vi "stft_demodulate_low.vi"(6 "Reset":bool, 9 "Config":T3={"IO params"={"Conversion"={"Rate"=4.0, "Num cards"=2, "Out channels"=4}, "Carriers"={"Phase shift"=180.0, "Levels"=[[0.8, 0.8, 0.8], [0.03, 0.03, 0.03]], "Delay samples"=73.15}, "TCP"={"Host"="192.168.1.15", "Port"=6666, "Buffering"=6, "Timeout"=6}, "Input channel sign"=[1, 1, 1]}, "High rate STFT"={"Win param"=101.5, "Window type"=61, "Win order"=2, "DFT size"=64, "Channels"=[7], "Oversample"=64}, "Low rate STFT"={"Win param"=120.0, "Window type"=61, "Win order"=8, "DFT size"=64, "Channels"=[7], "Oversample"=64}, "Filtering "=[]} {"Filtering"."Distortion"."Limit" format="%#_3p"; "Filtering"."Distortion"."LF cut" format="%#_3p"; "Filtering"."Kalman"."Measure noise" format="%#_3p"; "Filtering"."Kalman"."Process noise" format="%#_3p"; "Filtering"."Hum"."Limit" format="%#_3p"; "Filtering"."Hum"."Frequency" format="%#_4p"; "Low rate STFT"."Oversample" min=1 step=1; "Low rate STFT"."Channels" min=0 step=1; "Low rate STFT"."DFT size" min=1 step=1; "Low rate STFT"."Window type" items=["Rectangle"=0, "Hanning"=1, "Hamming"=2, "Blackman-Harris"=3, "Exact Blackman"=4, "Blackman"=5, "Flat Top"=6, "4 Term B-Harris "=7, "7 Term B-Harris"=8, "Low Sidelobe"=9, "Blackman Nuttall"=11, "Triangle"=30, "Bartlett-Hanning"=31, "Bohman"=32, "Parzen"=33, "Welch"=34, "Kaiser"=60, "Dolph-Chebyshev"=61, "Gaussian"=62]; "High rate STFT"."Oversample" min=1 step=1; "High rate STFT"."Channels" min=0 step=1; "High rate STFT"."DFT size" min=1 step=1; "High rate STFT"."Window type" items=["Rectangle"=0, "Hanning"=1, "Hamming"=2, "Blackman-Harris"=3, "Exact Blackman"=4, "Blackman"=5, "Flat Top"=6, "4 Term B-Harris "=7, "7 Term B-Harris"=8, "Low Sidelobe"=9, "Blackman Nuttall"=11, "Triangle"=30, "Bartlett-Hanning"=31, "Bohman"=32, "Parzen"=33, "Welch"=34, "Kaiser"=60, "Dolph-Chebyshev"=61, "Gaussian"=62]; "IO params"."Input channel sign" min=-1 max=1 step=1; "IO params"."Carriers"."Levels" min=0.0 step=0.1; "IO params"."Conversion"."Rate" format="%#_8g"}, 10 "Modulation info":T2={"Fs full"=0.0, "Fs high"=0.0, "Fs low"=0.0, "Read size"=0, "FFT size low"=5000, "df low"=5000.0, "High carriers"=[], "Low carriers"=[], "Hi channels at low"=[7]} {"Hi channels at low" min=0 step=1; "Low carriers" format="%#_6p"; "High carriers" format="%#_6p"}, 11 "Raw data":dbl[][](array[numeric])) -> (2 "STFT":cdb[][](array[numeric]) format="%#_4p", 3 "Card carrier amplitudes":T1 format="%#_3p")   [LabVIEW 2026]
uses:
  ilemt_config.ctl
  system/IO_params.ctl
  stft_params.ctl
  <vilib>/Analysis/4window.llb/windowTd.ctl
  filter_params.ctl
  detrend_mode.ctl
  modulation_info.ctl
  card_carrier_amplitudes.ctl
  <vilib>/Analysis/NI_AALPro.lvlib
panel:
  # "The demodulated carrier amplitudes (a coupling matrix) . The page index is high/low."
  # "Each row is the complex spectrum for the XYZ input channels.  This gets stored in the trace info."
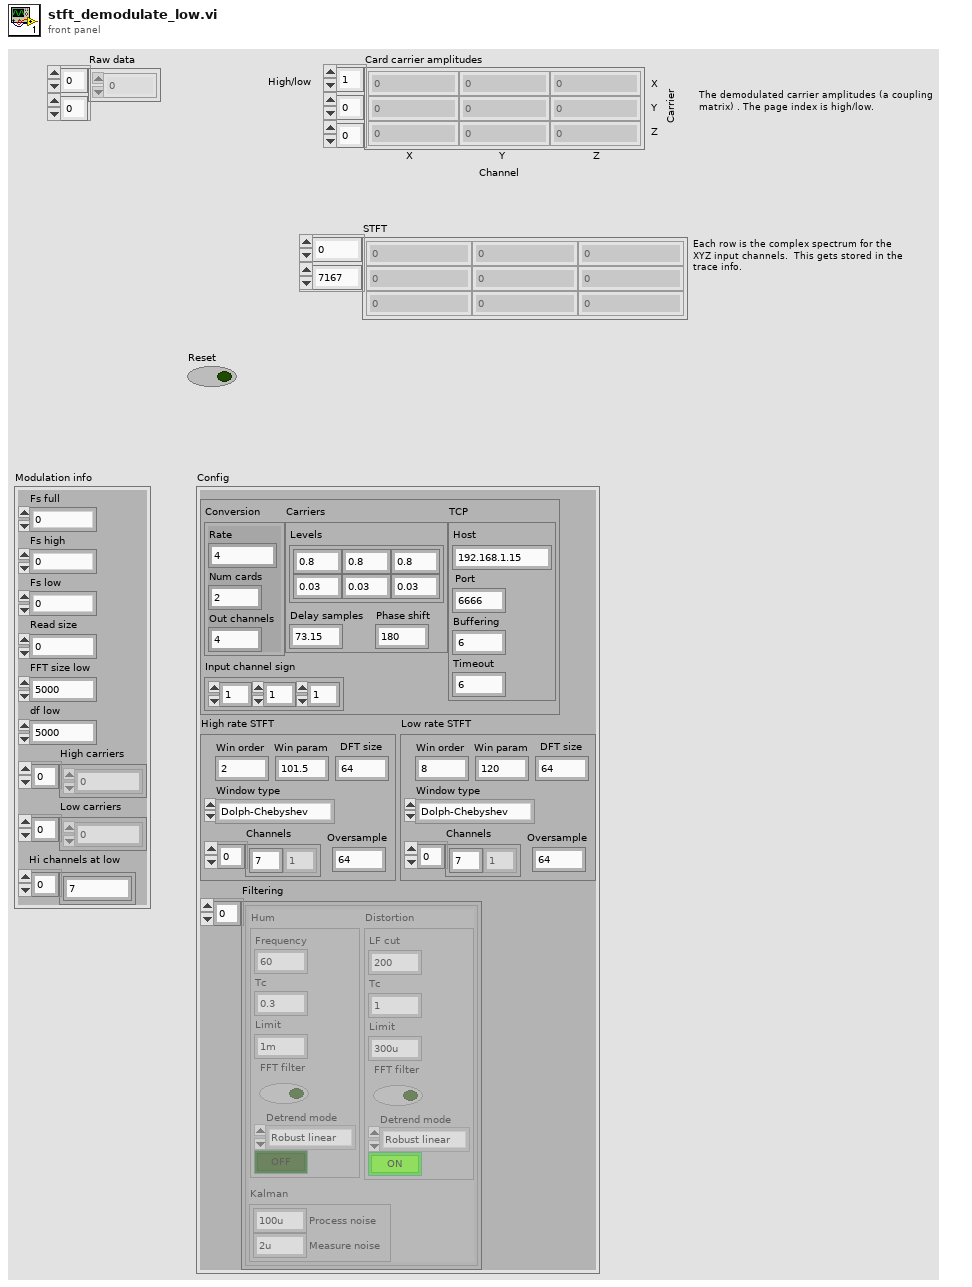
[diagram p1: front panel]
types:
  T1 = typedef "card_carrier_amplitudes.ctl" = cdb[][][]
  T2 = typedef "modulation_info.ctl" = cluster{"Fs full":dbl, "Fs high":dbl, "Fs low":dbl, "Read size":i32, "FFT size low":i32, "df low":dbl, "High carriers":dbl[], "Low carriers":dbl[], "Hi channels at low":i32[]}
  T3 = typedef "ilemt_config.ctl" = cluster{"IO params":T4, "High rate STFT":T5, "Low rate STFT":T5, "Filtering ":T7[]}
  T4 = typedef "IO_params.ctl" = cluster{"Conversion":cluster{"Rate":dbl, "Num cards":u32, "Out channels":u32}, "Carriers":cluster{"Phase shift":dbl, "Levels":dbl[][], "Delay samples":dbl}, "TCP":cluster{"Host":string, "Port":i32, "Buffering":u32, "Timeout":u32}, "Input channel sign":i32[]}
  T5 = typedef "stft_params.ctl" = cluster{"Win param":dbl, "Window type":T6, "Win order":i32, "DFT size":i32, "Channels":i32[], "Oversample":i32}
  T6 = typedef "NI_AALPro.lvlib/windowTd.ctl" = u32
  T7 = typedef "filter_params.ctl" = cluster{"Hum":cluster{"Frequency":dbl, "Tc":dbl, "Limit":dbl, "FFT filter":bool, "Detrend mode":T8, "Enable":bool}, "Kalman":cluster{"Process noise":dbl, "Measure noise":dbl}, "Distortion":cluster{"LF cut":dbl, "Tc":dbl, "Limit":dbl, "FFT filter":bool, "Detrend mode":T8, "Enable":bool}}
  T8 = typedef "detrend_mode.ctl" = enum16{"Zero mean", "Linear", "Robust linear"}
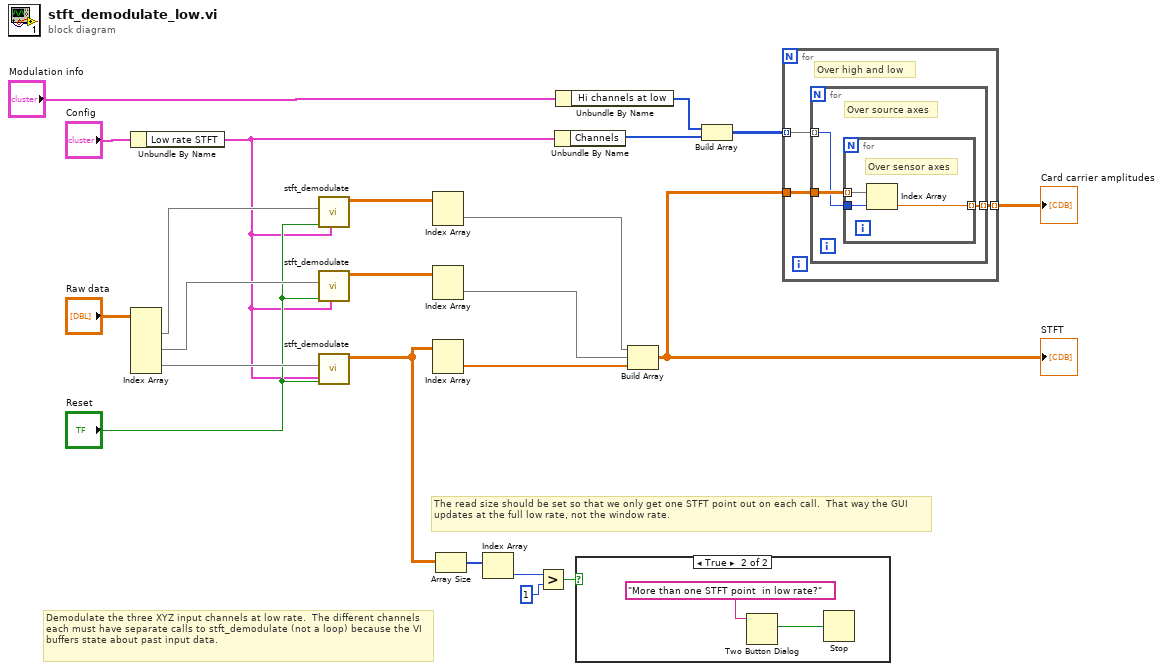
[diagram p0: block diagram]
diagram:
  # "Demodulate the three XYZ input channels at low rate.  The different channels each must have separate calls to stft_demodulate (not a loop) because the VI buffers state about past input data."
  # "The read size should be set so that we only get one STFT point out on each call.  That way the GUI updates at the full low rate, not the window rate."
  n1 = Unbundle By Name("Config") -> ("Low rate STFT"=w2:T5)
  n2 = Index Array(array="Raw data") -> (element #1=w9:dbl[], element #2=w14:dbl[], element #3=w16:dbl[])  [unwired: 6 in]
  n3 = call "stft_demodulate.vi"("STFT params"=w2, "Reset"="Reset", "X"=w9) -> ("STFT"=w13:cdb[][])  [unwired: 6 in, 2 out]
  n4 = call "stft_demodulate.vi"("STFT params"=w2, "Reset"="Reset", "X"=w14) -> ("STFT"=w12:cdb[][])  [unwired: 6 in, 2 out]
  n5 = call "stft_demodulate.vi"("STFT params"=w2, "Reset"="Reset", "X"=w16) -> ("STFT"=w18:cdb[][])  [unwired: 6 in, 2 out]
  n6 = Index Array(array=w13) -> (element=w11:cdb[])  [unwired: 2 in]
  n7 = Index Array(array=w12) -> (element=w10:cdb[])  [unwired: 2 in]
  n8 = Index Array(array=w18) -> (element=w17:cdb[])  [unwired: 2 in]
  n9 = Array Size(array=w18) -> (size(s)=w22:i32[])
  n10 = Index Array(array=w22) -> (element=w21:i32)  [unwired: 1 in]
  n11 = Greater?(x=w21, y=1 ("x")) -> (0:w19:bool)
  n12 = Unbundle By Name(w2) -> ("Channels"=w7:i32[])
  n13 = Unbundle By Name("Modulation info") -> ("Hi channels at low"=w6:i32[])
  n14 = case shown="True" w19 {
    frame False {
    }
    frame True {
      n15 = Two Button Dialog(message="More than one STFT point  in low rate?") -> (T button?=w24:bool)  [unwired: 2 in]
      n16 = Stop(stop? (T)=w24) -> ()
    }
  }
  n17 = Build Array(w11, w10, w17) -> (w4:cdb[][])
  "STFT" <- w4
  n18 = Build Array(w6, w7) -> (w5:i32[][])
  n19 = for {
    tunnel: w5 -> [w28] mode=indexing
    tunnel: [w27] -> w1 mode=indexing
    tunnel: w4 -> [w26]
    # "Over high and low"
    n20 = for {
      tunnel: w26 -> [w31]
      tunnel: w28 -> [w30] mode=indexing
      tunnel: [w29] -> w27 mode=indexing
      # "Over source axes"
      n21 = for {
        tunnel: w31 -> [w34] mode=indexing
        tunnel: w30 -> [w32]
        tunnel: [w33] -> w29 mode=indexing
        # "Over sensor axes"
        n22 = Index Array(array=w34, index=w32) -> (element=w33:cdb)
      }
    }
  }
  "Card carrier amplitudes" <- w1
